vi "Requests.vi"(8 "error in (no error)":errorcluster, 9 "write enable":bool=TRUE, 11 "ICPCON ET-7018i in":refnum<class "ICPCON ET-7018i.lvclass">) -> (0 "error out":errorcluster, 3 "ICPCON ET-7018i out":refnum<class "ICPCON ET-7018i.lvclass">)   [LabVIEW 2021, in "ICPCON ET-7018i.lvclass"]
uses:
  ICPCON ET-7018i.lvclass
  D:/my_projects/projects/Algorithms/Labview/21/Master CR/Master CR.lvclass
  D:/my_projects/projects/Algorithms/Labview/21/Master CR/Devices/ET7000/TCP/TCP.lvclass
  Master CR.lvclass/Master CR.ctl
  Modbus_v121c/Modbus Data Unit/Modbus Data Unit.lvclass/Modbus Data Unit.ctl
  Modbus_v121c/Network Protocol/Network Master/Network Master.lvclass/Network Master.ctl
  Modbus_v121c/Master Function Definition/Read Input Registers Request.vi
  Modbus_v121c/Master Function Definition/Read Input Registers Response.vi
  Modbus_v121c/Network Protocol/Network Master/Read write Master.vi
  Network Protocol/Read Network Protocol.vi
  Modbus_v121c/Modbus Data Unit/Construct PDU.vi
  Modbus_v121c/Utility/Bytes to U16s.vi
  Modbus_v121c/Master Function Definition/Function code mismatch error.vi
  Modbus_v121c/Data Model/Error Generator.vi
  Modbus_v121c/Modbus Data Unit/Deconstruct PDU.vi
  TCP/TCP.lvclass
  Modbus_v121c/Network Protocol/Network Master/Network Master.lvclass
  Modbus_v121c/Modbus Data Unit/Modbus Data Unit.lvclass
  Modbus_v121c/Data Model/Device Data Model.lvclass
  Modbus_v121c/Transmission Data Unit/Transmission Data Unit.lvclass
  Master CR.lvclass
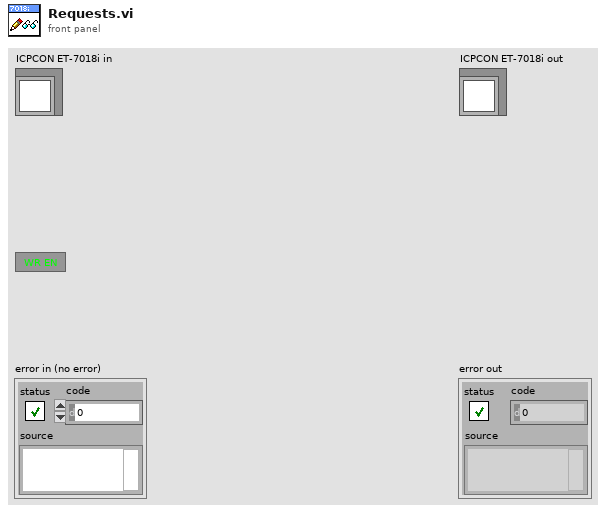
[diagram p1: front panel]
types:
  T1 = typedef "Device Data Model.lvclass/N channel.ctl" = cluster{"N DI channel":i32, "N DO channel":i32, "N AI channel":i32, "N AO channel":i32}
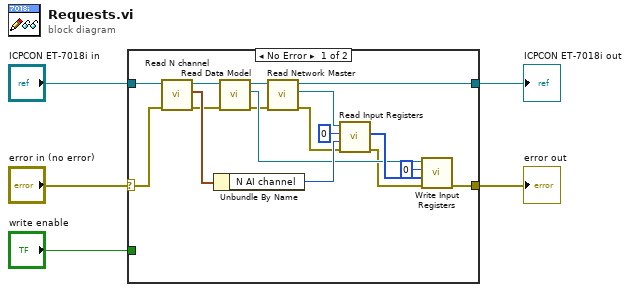
[diagram p0: block diagram]
diagram:
  n1 = case shown="No Error" "error in (no error)" {
    selector: "error in (no error)" -> [w15 w24]
    tunnel: [w11 w24] -> w3
    tunnel: [w6 w23] -> w2
    tunnel: "ICPCON ET-7018i in" -> [w17 w23]
    tunnel: "write enable" -> [_ _]
    frame No Error {
      n2 = call "Read N channel.vi"("error in (no error)"=w15, "Master CR in"=w17) -> ("error out"=w14:errorcluster, "N channel"=w19:T1, "Master CR out"=w16:refnum<class "ICPCON ET-7018i.lvclass">)  [unwired: 7 in]
      n3 = Unbundle By Name(w19) -> ("N AI channel"=w18:i32)
      n4 = call "Read Data Model.vi"("error in (no error)"=w14, "Master CR in"=w16) -> ("error out"=w10:errorcluster, "Data Model"=w13:refnum<class "Device Data Model.lvclass">, "Master CR out"=w9:refnum<class "ICPCON ET-7018i.lvclass">)  [unwired: 7 in]
      n5 = call "Read Network Master.vi"("error in (no error)"=w10, "TCP in"=w9) -> ("error out"=w7:errorcluster, "Network Master"=w8:refnum<class "Network Master.lvclass">, "TCP out"=w6:refnum<class "ICPCON ET-7018i.lvclass">)  [unwired: 7 in]
      n6 = call "Read Input Registers.vi"("error in (no error)"=w7, "number of input registers"=w18, "starting address"=u16 0, "Modbus master in"=w8) -> ("error out"=w12:errorcluster, "register values"=w21:u16[])  [unwired: 5 in, 1 out]
      n7 = call-dynamic "Write Input Registers.vi"("error in (no error)"=w12, "register values"=w21, "starting address"=u16 0, "Device Data Model in"=w13) -> ("error out"=w11:errorcluster)  [unwired: 6 in, 1 out]
    }
    frame Error {
    }
  }
  "error out" <- w3
  "ICPCON ET-7018i out" <- w2
